vi "ExDataCollectFocusImage.vi"() -> ()   [LabVIEW 2010]
uses:
  Open-Close Hardware/CamHandle.vi
panel:
  in  "Display Divider":i32=2
  in  "Stop collection":bool
  out "ready to \nstart":bool
  in  "Start collection":bool
  in  "Exposure":dbl=0.004 min=0.0 step=0.001 format="%.3f"
  out "error out":errorcluster
  in  "error in (no error)":errorcluster
  # "ExDataCollectFocusImage:\nthis example collects data for Image.\nRun this vi and wait for the ready to start to turn green.\nThen hit the start button to collect and display the image in separate image display window."
  # "1 - good for small images\n2 - good for normal images like 1024 x 1024\n3 - good for images > 1024 x 1024\n4 - good for images 2048 x 2048"
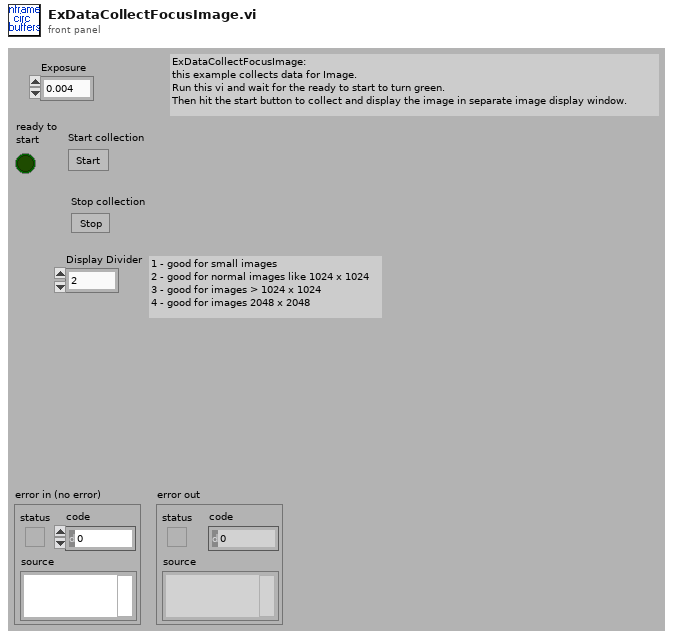
[diagram p1: front panel]
types:
  T1 = cluster{"Camera Handle":u32, "Pulser Handle":u32, "File Handle":u32, "Display Handle":u32, "Image Handle":u32}
  T2 = cluster{"acquire focus mode":u32, "Exposure":dbl, i32, "Software accumulation":u32}
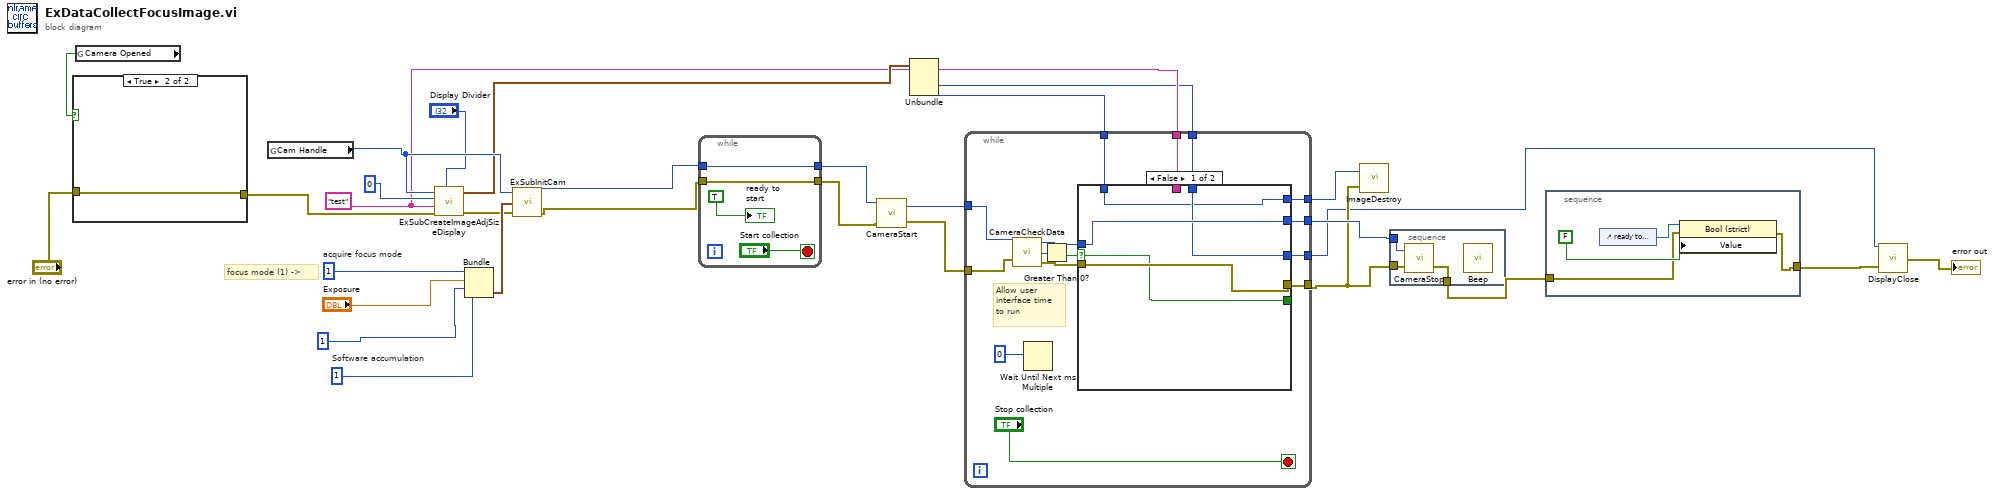
[diagram p0: block diagram]
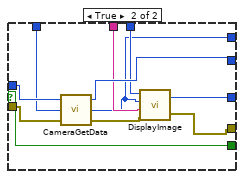
[diagram p2: hidden frame]
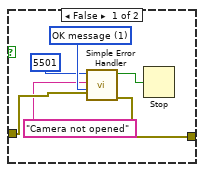
[diagram p3: hidden frame]
diagram:
  w9 = "test"
  w27 = u32 1  # acquire focus mode
  w26 = u32 1  # Software accumulation
  # "focus mode (1) ->"
  n1 = global read "CamHandle.vi" "Camera Opened"() -> (w24:bool)
  n2 = case shown="True" w24 {
    tunnel: "error in (no error)" -> [w34 w36]
    tunnel: [w33 w36] -> w19
    frame False {
      w35 = u16 1 items=["no dialog", "OK message", "continue or stop message"] ("type of dialog (OK msg:1)")
      n3 = call <vilib>:"Simple Error Handler.vi"("error code (no error:0)"=5501, "error source (\" \")"="Camera not opened", "type of dialog (OK msg:1)"=w35, "error in (no error)"=w34) -> ("error?"=w31:bool, "error out"=w33:errorcluster)  [unwired: 1 in, 3 out]
      n4 = Stop(stop? (T)=w31) -> ()
    }
    frame True {
    }
  }
  n5 = global read "CamHandle.vi" "Cam Handle"() -> (w13:u32)
  n6 = call "ExSubCreateImageAdjSizeDisplay.vi"("Camera Handle"=w13, "Pulser Handle"=0, "File and Display Name"=w9, "error in (no error)"=w19, "divider"="Display Divider") -> ("Handles Out"=w11:T1, "error out"=w18:errorcluster)  [unwired: 1 in]
  n7 = Bundle("acquire focus mode"=w27, "Exposure"="Exposure", 1, "Software accumulation"=w26) -> (w28:T2)  [unwired: 1 in]
  n8 = call "ExSubInitCam.vi"("error in (no error)"=w18, "Camera Information"=w28, "Camera Handle"=w13) -> ("error out"=w2:errorcluster, "Camera Handle"=w3:u32)
  n9 = while {
    tunnel: w2 -> [w38]
    tunnel: [w38] -> w23
    tunnel: w3 -> [w37]
    tunnel: [w37] -> w22
    stop <- "Start collection" stop-if-true
    "ready to \nstart" <- TRUE
  }
  n10 = call <userlib>:"CameraStart.vi"("error in"=w23, "Camera Handle"=w22) -> ("error out"=w20:errorcluster, "Camera Handle"=w21:u32)
  n11 = Unbundle(w11) -> ("Display Handle"=w8:u32, "Image Handle"=w10:u32)  [unwired: 3 out]
  n12 = while {
    tunnel: w21 -> [w51]
    tunnel: w20 -> [w50]
    tunnel: [w48] -> w15
    tunnel: [w47] -> w17
    tunnel: w10 -> [w42]
    tunnel: w9 -> [w46]
    tunnel: w8 -> [w45]
    tunnel: [w44] -> w5
    tunnel: [w43] -> w4
    stop <- "Stop collection" stop-if-true
    # "Allow user \ninterface time\nto run"
    n13 = call <userlib>:"CameraCheckData.vi"("Camera Handle"=w51, "error in"=w50) -> ("Camera Handle"=w53:u32, "Number Of Frames Available"=w55:i32, "error out"=w52:errorcluster)
    n14 = Wait Until Next ms Multiple(millisecond multiple=0) -> ()  [unwired: 1 out]
    n15 = Greater Than 0?(x=w55) -> (x > 0?=w54:bool)
    n16 = case shown="False" w54 {
      selector: w54 -> [w59 w69]
      tunnel: w53 -> [w58 w71]
      tunnel: w52 -> [w60 w70]
      tunnel: [w59 w69] -> _
      tunnel: [w60 w66] -> w48
      tunnel: [w58 w68] -> w47
      tunnel: w46 -> [_ w64]
      tunnel: w45 -> [w57 w63]
      tunnel: [w57 w62] -> w44
      tunnel: [w56 w61] -> w43
      tunnel: w42 -> [w56 w67]
      frame False {
      }
      frame True {
        n17 = call <userlib>:"CameraGetData.vi"("error in"=w70, "Data Handle"=w67, "Camera Handle"=w71) -> ("error out"=w65:errorcluster, "Data Handle"=w61:u32, "Camera Handle"=w68:u32)
        n18 = call <userlib>:"DisplayImage.vi"("error in"=w65, "Title"=w64, "Image Handle"=w61, "Display Handle"=w63) -> ("error out"=w66:errorcluster, "Display Handle"=w62:u32)
      }
    }
  }
  n19 = call <userlib>:"ImageDestroy.vi"("error in"=w15, "Data handle"=w4) -> ()  [unwired: 1 out]
  n20 = stacked-sequence {
    tunnel: w17 -> [w74]
    tunnel: [w73] -> w16
    tunnel: w15 -> [w72]
    frame #0 {
      n21 = call <userlib>:"CameraStop.vi"("error in"=w72, "Camera Handle"=w74) -> ("error out"=w73:errorcluster)  [unwired: 1 out]
      n22 = call <vilib>:"Beep.vi"() -> ()  [unwired: 12 in]
    }
  }
  n23 = stacked-sequence {
    tunnel: [w76] -> w7
    tunnel: w16 -> [w75]
    frame #0 {
      n24 = control-ref of="ready to \nstart"() -> (w78:refnum<vi>)
      n25 = property class="Bool (strict)"(reference=w78, error in=w75, "Value"=FALSE) -> (error out=w76:errorcluster)  [unwired: 1 out]
    }
  }
  n26 = call <userlib>:"DisplayClose.vi"("error in"=w7, "Display Handle"=w5) -> ("error out"=→"error out":errorcluster)
